vi "Write Font, Size & Style.vi"(8 "error in (no error)":errorcluster, 10 "Font, Size & Style":T1={"Desired Font (Application)"=enum."User-specified Font", "[User-specified Font]"={"Font Name"="Arial", "Size"=100, "Strikeout?"=FALSE, "Italic?"=FALSE, "Underline?"=FALSE, "Outline?"=FALSE, "Shadow?"=FALSE, "Bold?"=TRUE, "Rotation Angle"=0.0}, "Horizontal Alignment"=0, "Vertical Alignment"=0} {"Vertical Alignment" items=["Bottom", "Top", "Baseline"]; "Horizontal Alignment" items=["Left", "Center", "Right"]; "[User-specified Font]"."Rotation Angle" format="%.2f"}, 11 "Overlay Base in":refnum<class "Analyze Results Base.lvclass">) -> (0 "error out":errorcluster, 3 "Overlay Base out":refnum<class "Analyze Results Base.lvclass">)   [LabVIEW 2014, in "Analyze Results Base.lvclass"]
uses:
  Analyze Results Base.lvclass
  Analyze Results Base.lvclass/Analyze Results Base.ctl
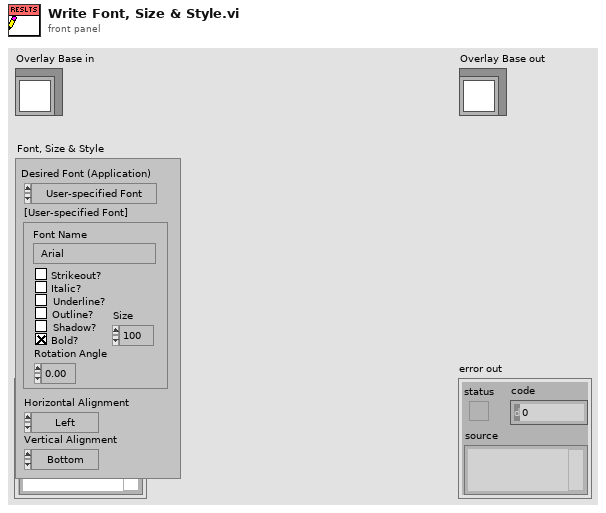
[diagram p1: front panel]
types:
  T1 = cluster{"Desired Font (Application)":enum16{"User-specified Font", "Application Font", "System Font", "Dialog Font"}, "[User-specified Font]":cluster{"Font Name":string, "Size":i16, "Strikeout?":bool, "Italic?":bool, "Underline?":bool, "Outline?":bool, "Shadow?":bool, "Bold?":bool, "Rotation Angle":dbl}, "Horizontal Alignment":i16, "Vertical Alignment":i16}
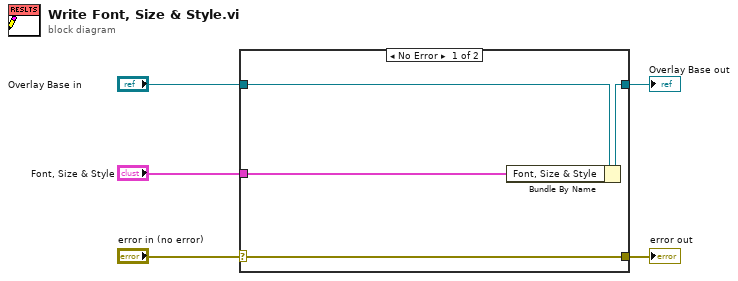
[diagram p0: block diagram]
diagram:
  n1 = case shown="No Error" "error in (no error)" {
    selector: "error in (no error)" -> [w9 w10]
    tunnel: [w9 w10] -> w4
    tunnel: [w7 w11] -> w2
    tunnel: "Overlay Base in" -> [w8 w11]
    tunnel: "Font, Size & Style" -> [w6 _]
    frame No Error {
      n2 = Bundle By Name(cluster=w8, "Font, Size & Style"=w6) -> (w7:refnum<class "Analyze Results Base.lvclass">)
    }
    frame Error {
    }
  }
  "error out" <- w4
  "Overlay Base out" <- w2
